vi "Csv.vi"(10 "Delayed RMS2>RMS1 for 3 data":dynamicdata(waveform), 11 "Byte Stream File in":refnum<file>) -> (3 "Byte Stream File out":refnum<file>)   [LabVIEW 2021]
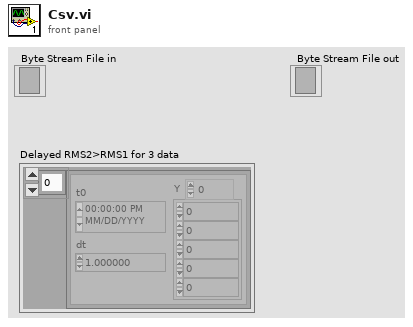
[diagram p1: front panel]
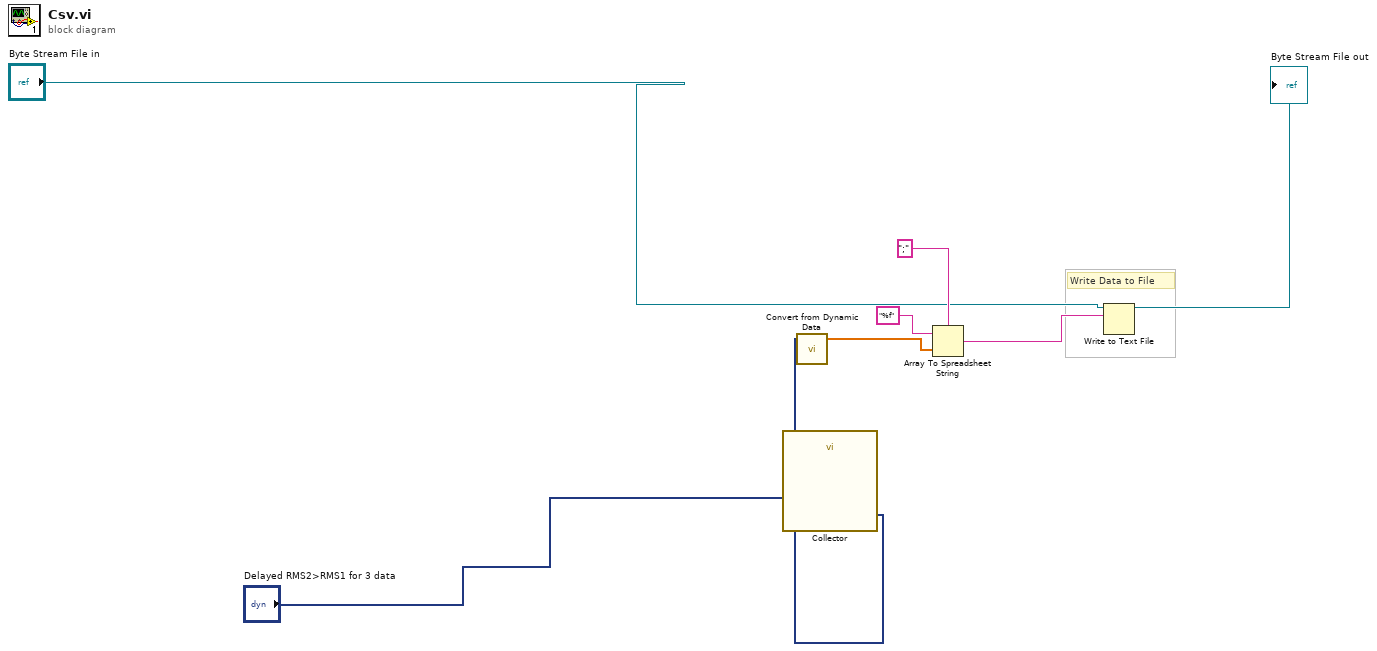
[diagram p0: block diagram]
diagram:
  # "Write Data to File"
  n1 = call "Collector"("Signals"="Delayed RMS2>RMS1 for 3 data") -> ("Collected Signals"=w1:dynamicdata)  [unwired: 9 in, 1 out]
  n2 = call "Convert from Dynamic Data"("Dynamic Data Type"=w1) -> ("Array"=w3:dbl[])  [unwired: 3 in]
  n3 = Array To Spreadsheet String(delimiter (Tab)=";" ("delimiter (\\t)"), array=w3, 3:"%f" ("format string")) -> (spreadsheet string=w4:string)
  n4 = Write to Text File(file (use dialog)="Byte Stream File in", text=w4) -> (refnum out=→"Byte Stream File out":refnum<file>)  [unwired: 2 in, 2 out]
